vi "Max Read Single.vi"(8 "error in":errorcluster, 9 "Channel Index":i32=1, 11 "Max Pressure Limit in":refnum<class "Pressure Limit.lvclass">) -> (0 "error out":errorcluster, 1 "Changed or First Call?":bool, 2 "Pressure Max SP":dbl, 3 "Max Pressure Limit out":refnum<class "Pressure Limit.lvclass">)   [LabVIEW 2023, in "Pressure Limit.lvclass"]
uses:
  Pressure Limit.lvclass
  Pressure Limit.lvclass/Pressure Limit.ctl
  Parents/Limit/Limit.lvclass
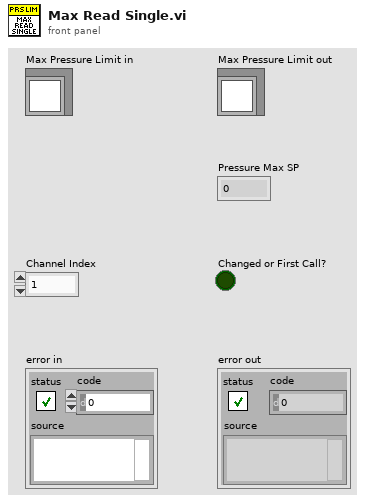
[diagram p1: front panel]
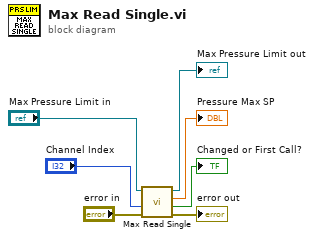
[diagram p0: block diagram]
diagram:
  n1 = call-parent "Max Read Single.vi"("error in"="error in", "Channel Index"="Channel Index", "Max Limit in"="Max Pressure Limit in") -> ("error out"=→"error out":errorcluster, "Changed or First Call?"=→"Changed or First Call?":bool, "Current Max SP"=→"Pressure Max SP":dbl, "Max Limit out"=→"Max Pressure Limit out":refnum<class "Pressure Limit.lvclass">)  [unwired: 5 in]
